vi "Scale Max and Min (SubVI).vi"(8 "error in (no error)":errorcluster, 11 "Scale":tag) -> (0 "error out":errorcluster, 2 "Max":dbl, 3 "Min":dbl)   [LabVIEW 2011]
uses:
  Program Files (x86)/National Instruments/LabVIEW 2011/resource/objmgr/daqmx.rc
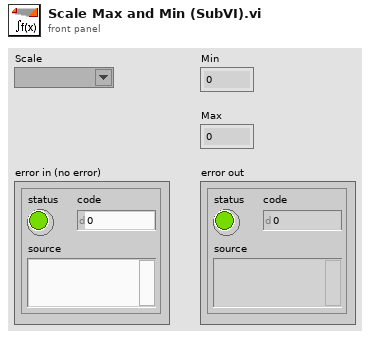
[diagram p1: front panel]
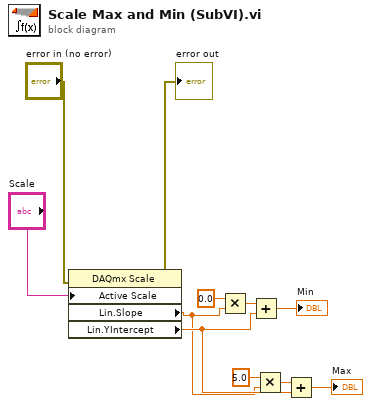
[diagram p0: block diagram]
diagram:
  n1 = property class="DAQmx Scale"(error in="error in (no error)", "Active Scale"="Scale") -> (error out=→"error out":errorcluster, "Lin.Slope"=w6:dbl, "Lin.YIntercept"=w7:dbl)  [unwired: 1 in, 1 out]
  n2 = Multiply(x=0.0, y=w6) -> (x*y=w2:dbl)
  n3 = Add(x=w2, y=w7) -> (x+y=→"Min":dbl)
  n4 = Multiply(x=5.0, y=w6) -> (x*y=w4:dbl)
  n5 = Add(x=w4, y=w7) -> (x+y=→"Max":dbl)
